vi "verify user login.vi"(6 "Required Permisions":T4, 7 "ENV":T2, 8 "error in (no error)":errorcluster, 9 "Settings":T1, 10 "POST Data (\"\")":string, 11 "Connection Refnum":T3) -> (0 "error out":errorcluster, 1 "User Verified\nand Spartan\nAuthorized?":bool, 2 "Response Header":string, 3 "dup Connection Refnum":T3, 4 "User":T4, 5 "updated ENV":T2)   [LabVIEW 2011]
uses:
  server/database/Users/User Record.ctl
  Addons/internet/utils/keyedarr.llb/Keyed Array.ctl
  SI.LIB/ODBC/SQL Controls/Connection Refnum.ctl
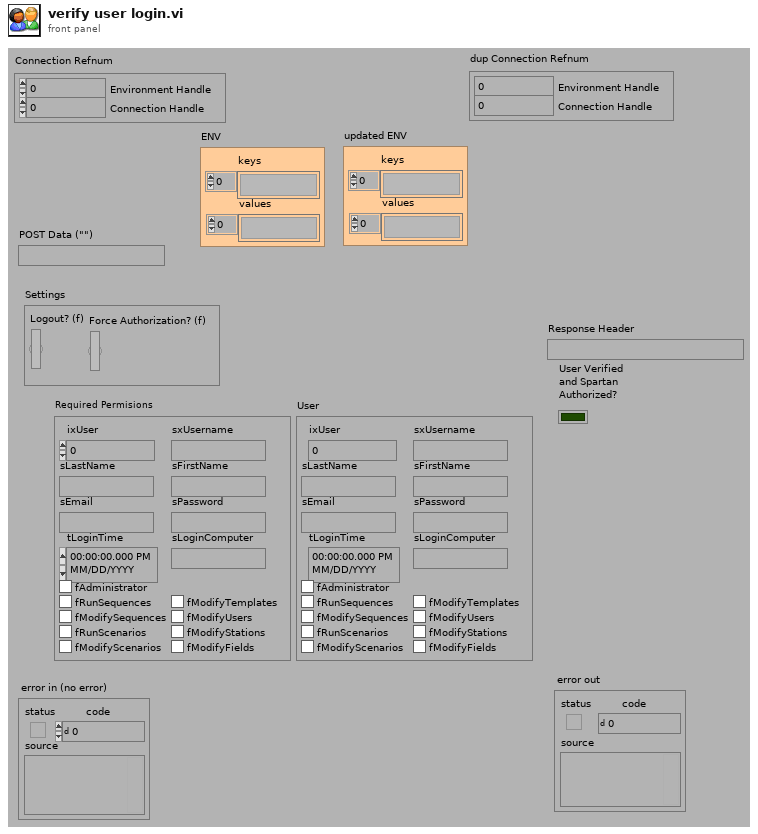
[diagram p1: front panel]
types:
  T1 = cluster{"Logout? (f)":bool, "Force Authorization? (f)":bool}
  T2 = typedef "Keyed Array.ctl" = cluster{"keys":string[], "values":string[]}
  T3 = typedef "Connection Refnum.ctl" = cluster{"Environment Handle":i32, "Connection Handle":i32}
  T4 = typedef "User Record.ctl" = cluster{"ixUser":i32, "sxUsername":string, "sLastName":string, "sFirstName":string, "sEmail":string, "sPassword":string, "tLoginTime":timestamp, "sLoginComputer":string, "fAdministrator":bool, "fRunSequences":bool, "fModifySequences":bool, "fRunScenarios":bool, "fModifyScenarios":bool, "fModifyTemplates":bool, "fModifyUsers":bool, "fModifyStations":bool, "fModifyFields":bool}
  T5 = typedef "Authorization Data.ctl" = cluster{"Valid":bool, "Seats":i32, "Expire Time":timestamp, "Last Access Time":timestamp, "Product ID":string, "Hardware ID":string, "Spartan Serial Number":string, "Feature":cluster{"#attributes":cluster{"Name":string, "Value":string}}[]}
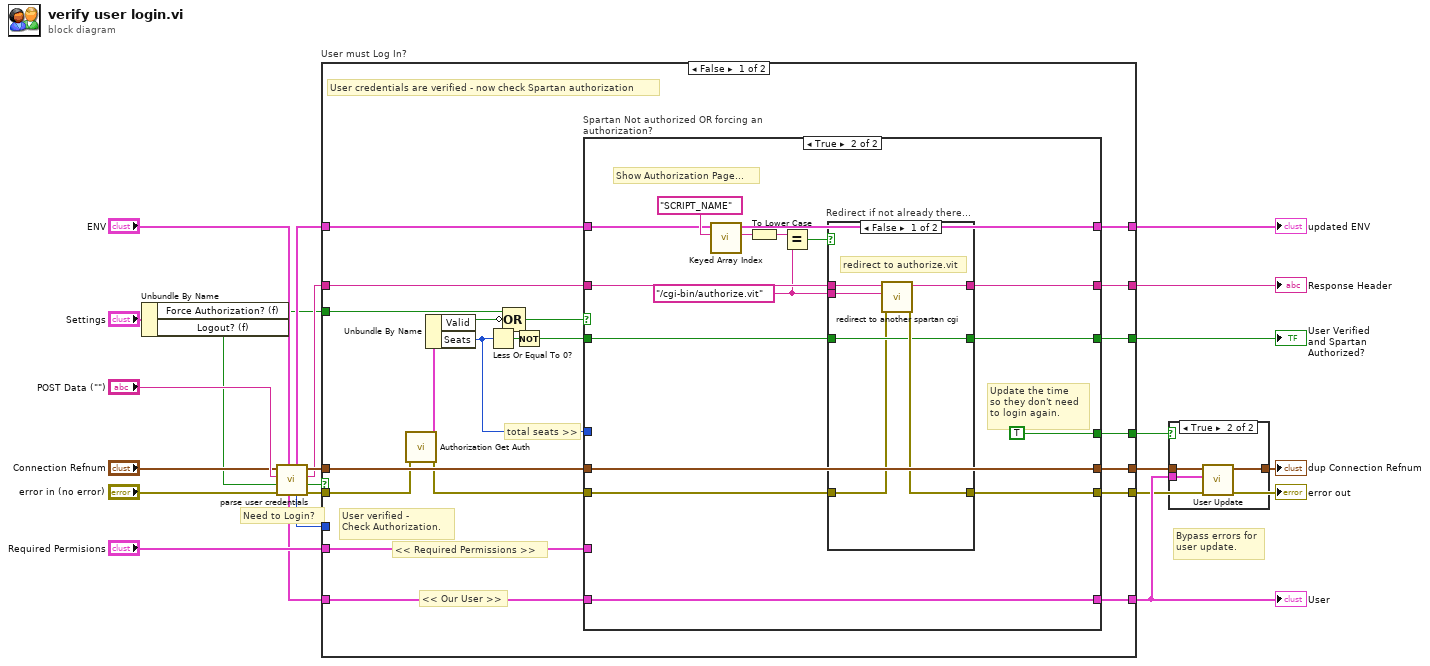
[diagram p0: block diagram]
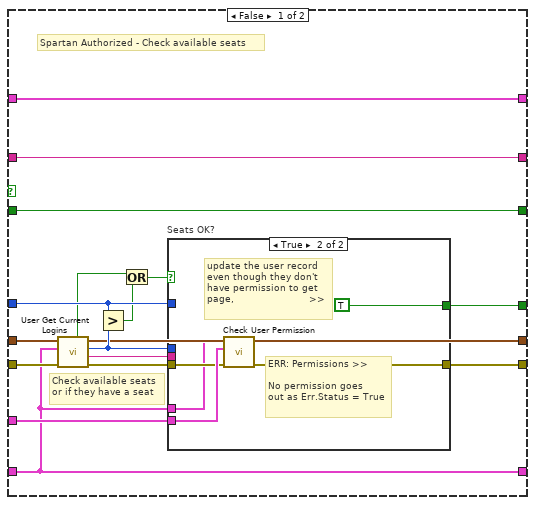
[diagram p3: hidden frame]
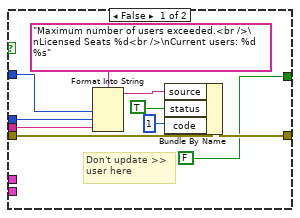
[diagram p4: hidden frame]
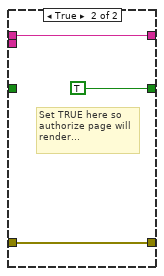
[diagram p5: hidden frame]
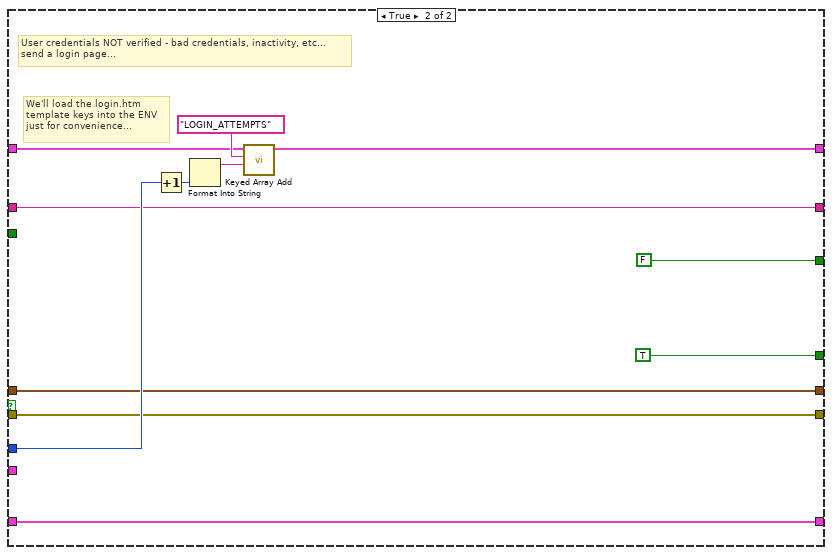
[diagram p6: hidden frame]
diagram:
  # "Bypass errors for\nuser update."
  # "Need to Login?"
  n1 = Unbundle By Name("Settings") -> ("Force Authorization? (f)"=w3:bool, "Logout? (f)"=w2:bool)
  n2 = call "parse user credentials.vi"("ENV"="ENV", "error in (no error)"="error in (no error)", "Logout? (f)"=w2, "Post Data (\"\")"="POST Data (\"\")", "Connection Refnum"="Connection Refnum") -> ("error out"=w17:errorcluster, "Login?"=w19:bool, "Response Header"=w5:string, "dup Connection Refnum"=w16:T3, "attempts"=w18:i32, "updated ENV"=w6:T2, "User"=w8:T4)
  n3 = case "User must Log In?" shown="False" w19 {
    tunnel: [w44 w102] -> w12
    tunnel: w17 -> [w28 w102]
    tunnel: w6 -> [w32 w104]
    tunnel: w5 -> [w43 w105]
    tunnel: [w42 w105] -> w23
    tunnel: [w34 FALSE] -> w21
    tunnel: "Required Permisions" -> [w41 _]
    tunnel: w8 -> [w40 w108]
    tunnel: [w39 w108] -> w13
    tunnel: w18 -> [_ w109]
    tunnel: w16 -> [w37 w106]
    tunnel: [w36 w106] -> w15
    tunnel: [w31 TRUE] -> w14
    tunnel: w3 -> [w30 _]
    tunnel: [w29 w103] -> w7
    frame False {
      # "total seats >>"
      # "<< Our User >>"
      # "User credentials are verified - now check Spartan authorization"
      # "<< Required Permissions >>"
      # "User verified - \nCheck Authorization."
      n4 = call "Authorization Get Auth.vi"("error in (no error)"=w28) -> ("error out"=w27:errorcluster, "Authorization"=w26:T5)  [unwired: 9 in]
      n5 = Unbundle By Name(w26) -> ("Valid"=w24:bool, "Seats"=w25:i32)
      n6 = Less Or Equal To 0?(x=w25) -> (x <= 0?=w33:bool)
      n7 = Compound Arithmetic op=OR(w30, invert w24, w33) -> (w38:bool)
      n8 = Not(x=w33) -> (.not. x?=w35:bool)
      n9 = case "Spartan Not authorized OR forcing an authorization?" shown="True" w38 {
        tunnel: w27 -> [w58 w82]
        tunnel: [w60 w80] -> w44
        tunnel: w43 -> [w61 w92]
        tunnel: [w61 w91] -> w42
        tunnel: w41 -> [w59 _]
        tunnel: w40 -> [w52 w90]
        tunnel: [w52 w90] -> w39
        tunnel: w37 -> [w53 w81]
        tunnel: [w46 w81] -> w36
        tunnel: w35 -> [w55 w85]
        tunnel: [w55 w84] -> w34
        tunnel: w25 -> [w54 _]
        tunnel: w32 -> [w45 w78]
        tunnel: [w47 TRUE] -> w31
        tunnel: [w45 w77] -> w29
        frame False {
          # "Spartan Authorized - Check available seats"
          # "Check available seats\nor if they have a seat"
          n10 = call "User Get Current Logins.vi"("error in (no error)"=w58, "Current User (none)"=w52, "Connection Refnum"=w53) -> ("error out"=w57:errorcluster, "Current User Summary"=w51:string, "Seats in Use"=w50:i32, "dup Connection Refnum"=w46:T3, "Current User has Seat?"=w49:bool)  [unwired: 1 in, 3 out]
          n11 = Greater?(x=w54, y=w50) -> (0:w48:bool)
          n12 = Or(x=w49, y=w48) -> (x .or. y?=w56:bool)
          n13 = case "Seats OK?" shown="True" w56 {
            tunnel: [w67 w73] -> w60
            tunnel: w59 -> [_ w76]
            tunnel: w57 -> [w64 w75]
            tunnel: w54 -> [w71 _]
            tunnel: w52 -> [_ w74]
            tunnel: w50 -> [w69 _]
            tunnel: w51 -> [w66 _]
            tunnel: [FALSE TRUE] -> w47
            frame False {
              # "Don't update >>\nuser here"
              n14 = Format Into String(format string="Maximum number of users exceeded.<br />\nLicensed Seats %d<br />\nCurrent users: %d %s", w71, w69, w66) -> (resulting string=w68:string)  [unwired: 2 in, 1 out]
              n15 = Bundle By Name(cluster=w64, "source"=w68, "status"=TRUE, "code"=1) -> (w67:errorcluster)
            }
            frame True {
              # "update the user record\neven though they don't\nhave permission to get\npage,                         >>"
              # "ERR: Permissions >>\n\nNo permission goes\nout as Err.Status = True"
              n16 = call "Check User Permission.vi"("error in"=w75, "Required Permisions"=w76, "User Record"=w74) -> ("error out"=w73:errorcluster)  [unwired: 8 out]
            }
          }
        }
        frame True {
          w87 = "/cgi-bin/authorize.vit" ("New URL (/cgi-bin/testing.vit)")
          # "Update the time\nso they don't need\nto login again."
          # "Show Authorization Page..."
          n17 = call "Keyed Array Index.vi"("key"="SCRIPT_NAME" ("New URL (/cgi-bin/testing.vit)"), "array in"=w78) -> ("value"=w88:string, "duplicate array"=w77:T2)  [unwired: 2 in, 2 out]
          n18 = To Lower Case(string=w88) -> (all lower case string=w83:string)
          n19 = Equal?(x=w83, y=w87) -> (x = y?=w86:bool)
          n20 = case "Redirect if not already there..." shown="False" w86 {
            tunnel: w92 -> [w98 w101]
            tunnel: [w97 w101] -> w91
            tunnel: w82 -> [w93 w100]
            tunnel: [w96 w100] -> w80
            tunnel: w87 -> [w95 _]
            tunnel: w85 -> [w94 _]
            tunnel: [w94 TRUE] -> w84
            frame False {
              # "redirect to authorize.vit"
              n21 = call "redirect to another spartan cgi.vi"("error in (no error)"=w93, "New URL (/cgi-bin/testing.vit)"=w95, "Original Header In (to be replaced)"=w98) -> ("error out"=w96:errorcluster, "Redirection Header"=w97:string)  [unwired: 1 in, 6 out]
            }
            frame True {
              # "Set TRUE here so\nauthorize page will\nrender..."
            }
          }
        }
      }
    }
    frame True {
      # "We'll load the login.htm\ntemplate keys into the ENV\njust for convenience..."
      # "User credentials NOT verified - bad credentials, inactivity, etc...\nsend a login page..."
      n22 = Increment(x=w109) -> (x+1=w111:i32)
      n23 = Format Into String(w111) -> (resulting string=w110:string)  [unwired: 3 in, 1 out]
      n24 = call "Keyed Array Add.vi"("value"=w110, "key"="LOGIN_ATTEMPTS", "array in"=w104) -> ("array out"=w103:T2)  [unwired: 1 in, 3 out]
    }
  }
  "error out" <- w12
  "Response Header" <- w23
  "User Verified\nand Spartan\nAuthorized?" <- w21
  "User" <- w13
  "updated ENV" <- w7
  n25 = case shown="True" w14 {
    tunnel: w15 -> [w114 w117]
    tunnel: w13 -> [_ w116]
    tunnel: [w114 w115] -> w1
    frame False {
    }
    frame True {
      n26 = call "User Update.vi"("User Record"=w116, "Connection Refnum"=w117) -> ("dup Connection Refnum"=w115:T3)  [unwired: 1 in, 8 out]
    }
  }
  "dup Connection Refnum" <- w1
